vi "test_Error Code Channel_Overwrite File If Exists Enabled.vi"(8 "error in (no error)":errorcluster, 11 "TestCase in":refnum<class "Telemetry System Tests.lvclass">=refnum) -> (0 "error out":errorcluster, 3 "TestCase out":refnum<class "Telemetry System Tests.lvclass">)   [LabVIEW 2026, in "Telemetry System Tests.lvclass"]
uses:
  Telemetry System Tests.lvclass
  b15e678b-00b4-460c-84a3-511904b6b81c.vi
  <vilib>/NI VeriStand/Execution/Workspace/NI_VS Workspace ExecutionAPI.lvlib
  <vilib>/NI VeriStand/Execution/Workspace/NI VeriStand - Get Single Channel Value.vi
  4f62a354-8c76-47c1-8a4a-adcdfc5b0832.vi
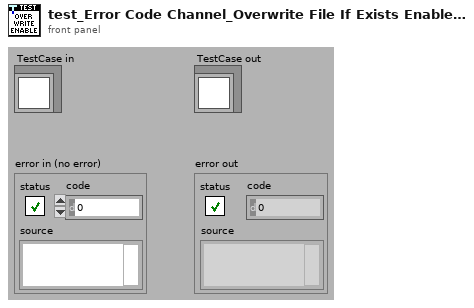
[diagram p1: front panel]
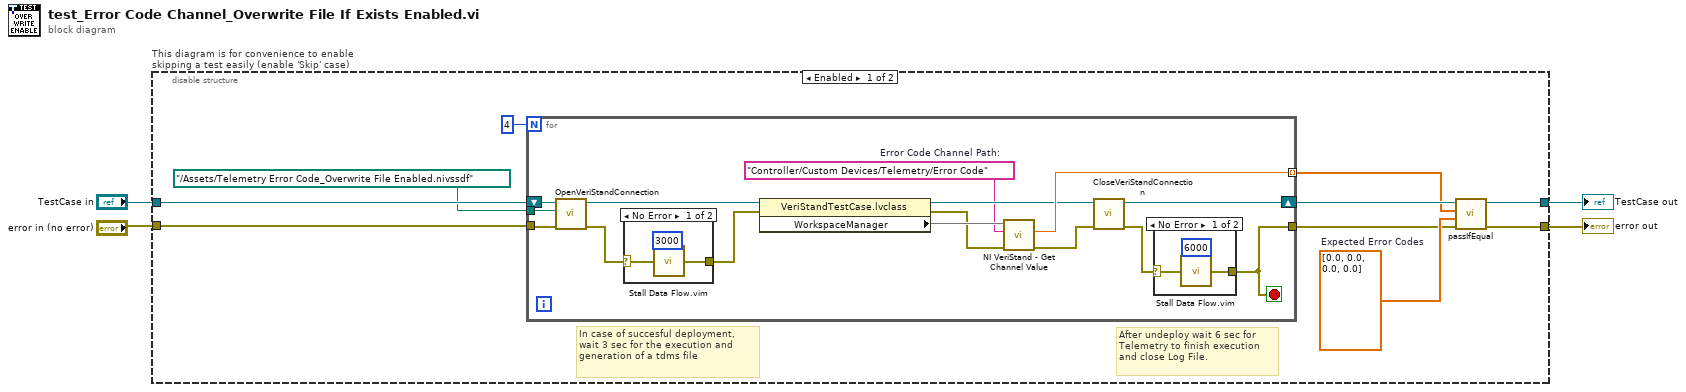
[diagram p0: block diagram]
diagram:
  n1 = disable-structure "This diagram is for convenience to enable skipping a test easily (enable 'Skip' case)" shown="Enabled" {
    disable-tunnel: "TestCase in" -> [w14 w41]
    disable-tunnel: [w7 w39] -> w1
    disable-tunnel: [w8 w40] -> w3
    disable-tunnel: "error in (no error)" -> [w5 w38]
    frame Enabled {
      w10 = dbl[] [0.0, 0.0, 0.0, 0.0]  # Expected Error Codes
      # "In case of succesful deployment, wait 3 sec for the execution and generation of a tdms file"
      # "After undeploy wait 6 sec for Telemetry to finish execution and close Log File."
      n2 = for {
        N: 4 -> [_]
        tunnel: w5 -> [w29]
        tunnel: path "../Assets/Telemetry Error Code_Overwrite File Enabled.nivssdf" ("System Definition File") -> [w26]
        shift-right: [w25] -> w13
        shift-left: w14 -> [w27]
        tunnel: [w23] -> w11 mode=indexing
        tunnel: [w16] -> w9
        stop <- w16 stop-if-true
        w17 = "Controller/Custom Devices/Telemetry/Error Code"  # Error Code Channel Path:
        n3 = call-dynamic "OpenVeriStandConnection.vi"("error in (no error)"=w29, "System Definition File"=w26, "VeriStand Test Case in"=w27) -> ("error out"=w28:errorcluster, "VeriStand Test Case out"=w21:refnum<class "VeriStandTestCase.lvclass">)  [unwired: 6 in, 1 out]
        n4 = case shown="No Error" w28 {
          selector: w28 -> [w36 w37]
          tunnel: [w34 w37] -> w22
          frame No Error {
            n5 = call "Stall Data Flow.vim"("value in"=w36, "milliseconds to wait"=u32 3000) -> ("value out"=w34:errorcluster)  [unwired: 1 out]
          }
          frame Error {
          }
        }
        n6 = property class="VeriStandTestCase.lvclass"(reference=w21, error in=w22) -> (reference out=w20:refnum<class "VeriStandTestCase.lvclass">, error out=w18:errorcluster, "WorkspaceManager"=w19)
        n7 = call-poly <vilib>:"NI VeriStand - Get Channel Value.vi"("error in (no error)"=w18, "Channel"=w17, "WorkspaceManager in"=w19) -> ("error out"=w24:errorcluster, "Value"=w23:dbl)  [unwired: 6 in, 1 out]
        n8 = call-dynamic "CloseVeriStandConnection.vi"("error in (no error)"=w24, "VeriStand Test Case in"=w20) -> ("error out"=w15:errorcluster, "VeriStand Test Case out"=w25:refnum<class "VeriStandTestCase.lvclass">)  [unwired: 8 in]
        n9 = case shown="No Error" w15 {
          selector: w15 -> [w30 w33]
          tunnel: [w32 w33] -> w16
          frame No Error {
            n10 = call "Stall Data Flow.vim"("value in"=w30, "milliseconds to wait"=u32 6000) -> ("value out"=w32:errorcluster)  [unwired: 1 out]
          }
          frame Error {
          }
        }
      }
      n11 = call-dynamic "passIfEqual.vi"("error in (no error)"=w9, "y"=w10, "x"=w11, "TestCase in"=w13) -> ("error out"=w8:errorcluster, "TestCase out"=w7:refnum<class "Telemetry System Tests.lvclass">)  [unwired: 6 in]
    }
    frame Disabled {
      # "skip test result while test is under development"
      n12 = call <vilib>:"skip.vi"("error in (no error)"=w38, "TestCase in"=w41) -> ("error out"=w40:errorcluster, "TestCase out"=w39:refnum<class "Telemetry System Tests.lvclass">)  [unwired: 8 in]
    }
  }
  "error out" <- w3
  "TestCase out" <- w1
